vi "Dashboard.vi"() -> ()   [LabVIEW 2025]
panel:
  out "bytes written":i32
  in  "mode (standard)":T1(ring)
  in  "remote port or service name":u16
  out "error out":errorcluster
  out "data out":string
  in  "stop":bool
  in  "timeout ms (60000)":i32=60000
  in  "address":string
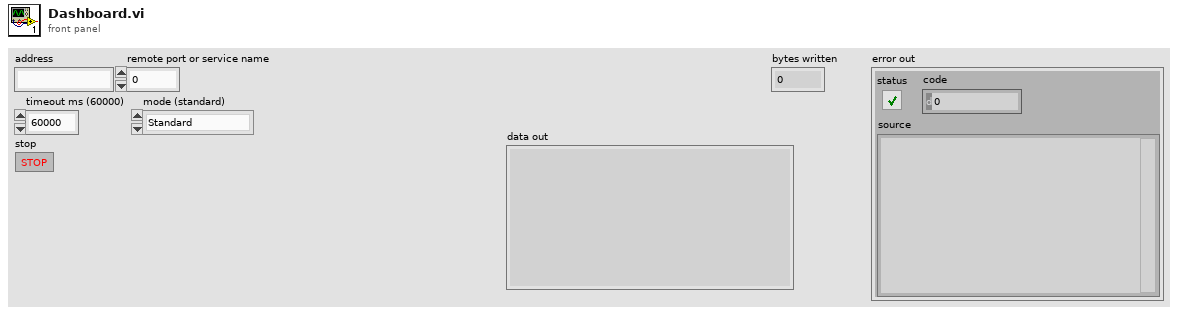
[diagram p1: front panel]
types:
  T1 = enum16{"Standard", "Buffered", "CRLF", "Immediate"}
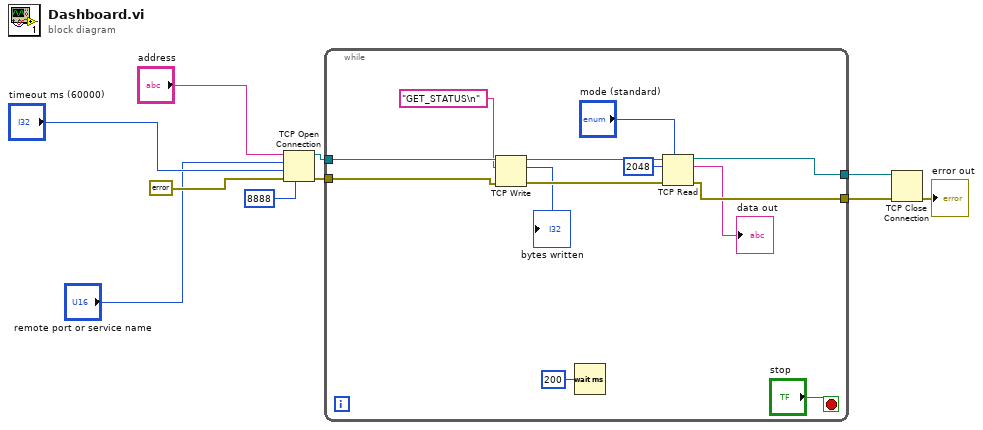
[diagram p0: block diagram]
diagram:
  n1 = TCP Open Connection(address="address", remote port or service name="remote port or service name", timeout ms (60000)="timeout ms (60000)", local port=u16 8888 ("local port (0)"), error in (no error)=errorcluster {"status"=FALSE, "code"=0, "source"=""}) -> (connection ID=w7:refnum<k5>, error out=w6:errorcluster)
  n2 = while {
    tunnel: w7 -> [w21]
    tunnel: w6 -> [w17]
    tunnel: [w16] -> w5
    tunnel: [w15] -> w4
    stop <- "stop" stop-if-true
    n3 = TCP Write(connection ID=w21, data in="GET_STATUS\n", error in (no error)=w17) -> (connection ID out=w19:refnum<k5>, bytes written=→"bytes written":i32, error out=w18:errorcluster)  [unwired: 1 in]
    n4 = Wait (ms)(milliseconds to wait=u32 200) -> ()  [unwired: 1 out]
    n5 = TCP Read(connection ID=w19, bytes to read=2048, error in (no error)=w18, 7:"mode (standard)") -> (connection ID out=w16:refnum<k5>, data out=→"data out":string, error out=w15:errorcluster)  [unwired: 1 in]
  }
  n6 = TCP Close Connection(connection ID=w5, error in (no error)=w4) -> (error out=→"error out":errorcluster)  [unwired: 1 in, 1 out]
